vi "Write Last Command Queue Time.vi"(8 "error in (no error)":errorcluster, 10 "Last Command Queue Time":timestamp, 11 "Command Processor Actor in":refnum<class "Command Processor Actor.lvclass">) -> (0 "error out":errorcluster, 3 "Command Processor Actor out":refnum<class "Command Processor Actor.lvclass">)   [LabVIEW 2014, in "Robot Actor Framework.lvlib" / "Command Processor Actor.lvlib" / "Command Processor Actor.lvclass"]
uses:
  Command Processor Actor.lvclass
  Command Processor Actor.lvclass/Command Processor Actor.ctl
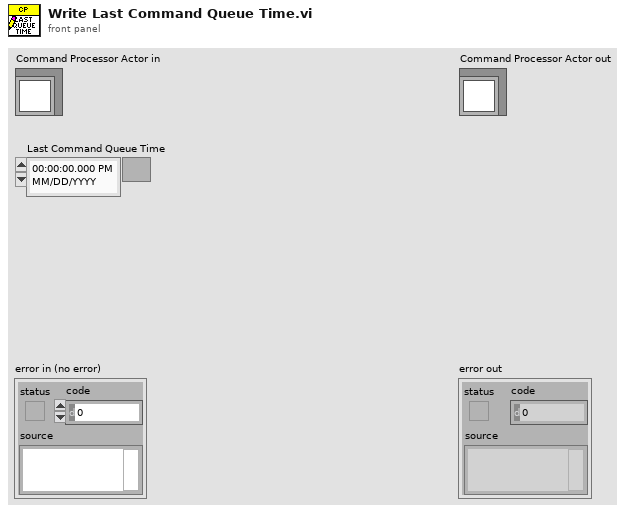
[diagram p1: front panel]
types:
  T1 = typedef "Robot Actor Framework.lvlib/Command Processor Actor.lvlib/Command Processor Actor.lvclass/Command Processor State.ctl" = cluster{"Current State":T2, "Last State Update":timestamp, "Queued Commands":u32, "Current Command Status":T3, "Previous State":T2, "Current State Entry":timestamp, "Transitioning State":bool, "Commands Behind":dbl, "Last Command Queue Time":timestamp}
  T2 = typedef "Robot Actor Framework.lvlib/Command Processor Actor.lvlib/Command Processor Actor.lvclass/Command Processor States.ctl" = enum16{"Unknown", "No Command", "Running Command", "Starting Command", "Stopping Command", "Finishing Command"}
  T3 = typedef "Robot Actor Framework.lvlib/Command Actor.lvlib/Command Actor.lvclass/Command State.ctl" = cluster{"Command Name":string, "Command Start Time":timestamp, "Command End Time":timestamp, "Is Command Finished?":bool, "Command ID":u32, "Command State":T4, "Command State Time":timestamp}
  T4 = typedef "Robot Actor Framework.lvlib/Command Actor.lvlib/Command Actor.lvclass/Command States.ctl" = enum16{"Unknown", "Started", "Stopped", "Finished"}
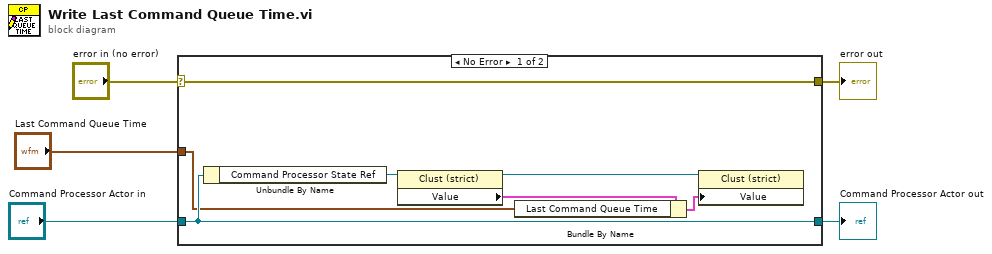
[diagram p0: block diagram]
diagram:
  n1 = case shown="No Error" "error in (no error)" {
    selector: "error in (no error)" -> [w12 w13]
    tunnel: [w12 w13] -> w4
    tunnel: [w11 w14] -> w2
    tunnel: "Command Processor Actor in" -> [w11 w14]
    tunnel: "Last Command Queue Time" -> [w6 _]
    frame No Error {
      n2 = Unbundle By Name(w11) -> ("Command Processor State Ref"=w10:refnum<vi>)
      n3 = property class="Clust (strict)"(reference=w10) -> (reference out=w9:refnum<vi>, "Value"=w8:T1)  [unwired: 1 in, 1 out]
      n4 = Bundle By Name(cluster=w8, "Last Command Queue Time"=w6) -> (w7:T1)
      n5 = property class="Clust (strict)"(reference=w9, "Value"=w7) -> ()  [unwired: 1 in, 2 out]
    }
    frame Error {
    }
  }
  "error out" <- w4
  "Command Processor Actor out" <- w2
